vi "Simulator PIM Preset.vi"(8 "error in (no error)":errorcluster, 11 "PIM Configuration":T1={"host IP (localhost)"="localhost", "host Port"=3388, "Model"="", "Serial Number(s)"="", "Calibration Date"=0.0, "Dual Port?"=FALSE, "DeviceNames"=[], "Parameters"={"TX1start"=0.0, "TX1stop"=0.0, "TX1pmax"=0.0, "TX2start"=0.0, "TX2stop"=0.0, "TX2pmax"=0.0, "RXstart"=0.0, "RXstop"=0.0}, "Interface"=enum."PIM Web Engine"} {"Calibration Date" format="%.2f"; "Parameters"."TX2pmax" format="%.1f"; "Parameters"."TX1pmax" format="%.1f"; "Parameters"."RXstop" format="%.1f"; "Parameters"."RXstart" format="%.1f"; "Parameters"."TX2stop" format="%.1f"; "Parameters"."TX2start" format="%.1f"; "Parameters"."TX1stop" format="%.1f"; "Parameters"."TX1start" format="%.1f"}) -> (0 "error out":errorcluster, 2 "Flattened TestSetDef w/Version":string, 3 "TestSetDef":T3={"General"={"ID"=0, "Model"="", "Dual Port?"=FALSE, "Options"="", "Options"={"E"=FALSE, "K"=FALSE, "H"=FALSE, "W"=FALSE, "F"=FALSE}, "Cal File"=path ""}, "Receiver"={"Fstart, MHz"=0.0, "Fstop MHz"=0.0, "Fstep MHz"=0.0, "IF, MHz"=0.0}, "RX Band"={"Fstart, MHz"=0.0, "Fstop MHz"=0.0}, "TX 1"={"Fstart, MHz"=0.0, "Fstop MHz"=0.0, "Pmax, dBm"=0.0, "Pstep, dB"=0.0}, "TX 2"={"Fstart, MHz"=0.0, "Fstop MHz"=0.0, "Pmax, dBm"=0.0, "Pstep, dB"=0.0}, "Low-side?"=TRUE})   [LabVIEW 2011]
uses:
  BPIMCore EXT/HW IO/Test Set Definition.ctl
  PIM Configuration.ctl
  PIM Interface Language.ctl
  Simulator PIM Version.vi
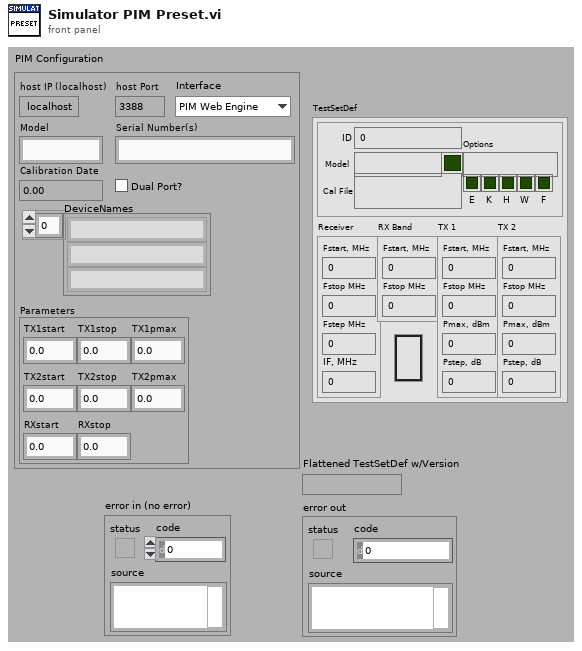
[diagram p1: front panel]
types:
  T1 = typedef "PIM Configuration.ctl" = cluster{"host IP (localhost)":string, "host Port":u16, "Model":string, "Serial Number(s)":string, "Calibration Date":dbl, "Dual Port?":bool, "DeviceNames":string[], "Parameters":cluster{"TX1start":dbl, "TX1stop":dbl, "TX1pmax":dbl, "TX2start":dbl, "TX2stop":dbl, "TX2pmax":dbl, "RXstart":dbl, "RXstop":dbl}, "Interface":T2}
  T2 = typedef "PIM Interface Language.ctl" = enum16{"PIM Web Engine", "PIM HW Engine"}
  T3 = typedef "Test Set Definition.ctl" = cluster{"General":cluster{"ID":u32, "Model":string, "Dual Port?":bool, "Options":string, "Options":cluster{"E":bool, "K":bool, "H":bool, "W":bool, "F":bool}, "Cal File":path}, "Receiver":cluster{"Fstart, MHz":dbl, "Fstop MHz":dbl, "Fstep MHz":dbl, "IF, MHz":dbl}, "RX Band":cluster{"Fstart, MHz":dbl, "Fstop MHz":dbl}, "TX 1":cluster{"Fstart, MHz":dbl, "Fstop MHz":dbl, "Pmax, dBm":dbl, "Pstep, dB":dbl}, "TX 2":cluster{"Fstart, MHz":dbl, "Fstop MHz":dbl, "Pmax, dBm":dbl, "Pstep, dB":dbl}, "Low-side?":bool}
  T4 = typedef "OGAB Version.ctl" = cluster{"Version":string, "Build Number":u32, "Build Date/Time":dbl}
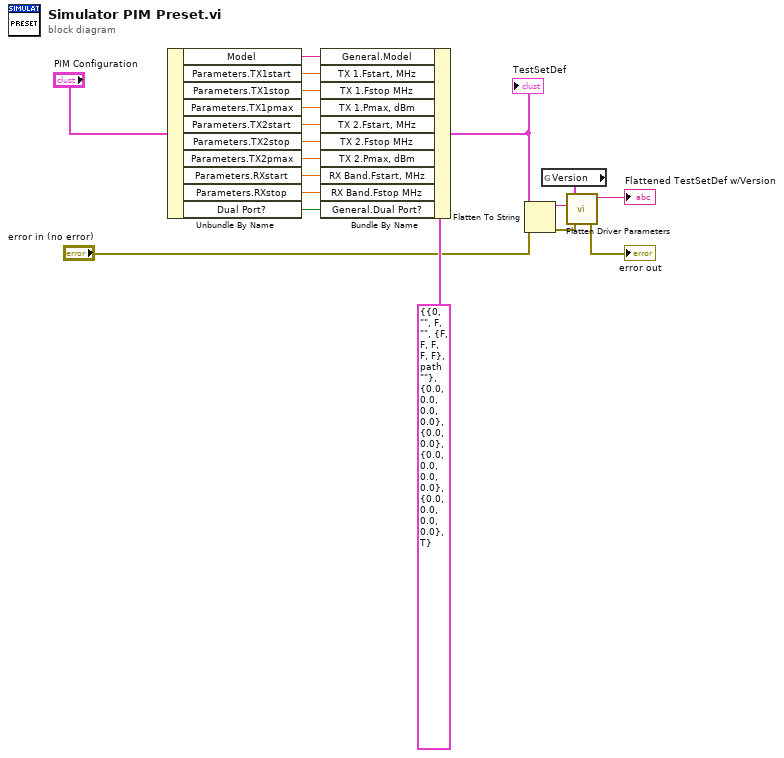
[diagram p0: block diagram]
diagram:
  n1 = Unbundle By Name("PIM Configuration") -> ("Model"=w12:string, "Parameters.TX1start"=w11:dbl, "Parameters.TX1stop"=w10:dbl, "Parameters.TX1pmax"=w9:dbl, "Parameters.TX2start"=w8:dbl, "Parameters.TX2stop"=w7:dbl, "Parameters.TX2pmax"=w6:dbl, "Parameters.RXstart"=w5:dbl, "Parameters.RXstop"=w4:dbl, "Dual Port?"=w1:bool)
  n2 = Bundle By Name(cluster=T3 {"General"={"ID"=0, "Model"="", "Dual Port?"=FALSE, "Options"="", "Options"={"E"=FALSE, "K"=FALSE, "H"=FALSE, "W"=FALSE, "F"=FALSE}, "Cal File"=path ""}, "Receiver"={"Fstart, MHz"=0.0, "Fstop MHz"=0.0, "Fstep MHz"=0.0, "IF, MHz"=0.0}, "RX Band"={"Fstart, MHz"=0.0, "Fstop MHz"=0.0}, "TX 1"={"Fstart, MHz"=0.0, "Fstop MHz"=0.0, "Pmax, dBm"=0.0, "Pstep, dB"=0.0}, "TX 2"={"Fstart, MHz"=0.0, "Fstop MHz"=0.0, "Pmax, dBm"=0.0, "Pstep, dB"=0.0}, "Low-side?"=TRUE} ("TestSetDef"), "General.Model"=w12, "TX 1.Fstart, MHz"=w11, "TX 1.Fstop MHz"=w10, "TX 1.Pmax, dBm"=w9, "TX 2.Fstart, MHz"=w8, "TX 2.Fstop MHz"=w7, "TX 2.Pmax, dBm"=w6, "RX Band.Fstart, MHz"=w5, "RX Band.Fstop MHz"=w4, "General.Dual Port?"=w1) -> (w3:T3)
  "TestSetDef" <- w3
  n3 = Flatten To String(anything=w3, error in (no error)="error in (no error)") -> (data string=w18:string, error out=w16:errorcluster)  [unwired: 3 out]
  n4 = global read "Simulator PIM Version.vi" "Version"() -> (w19:T4)
  n5 = call "Flatten Driver Parameters.vi"("error in (no error)"=w16, "Flattened Driver Parameters (\"\")"=w18, "Driver Version"=w19) -> ("error out"=→"error out":errorcluster, "Flattened Driver Parameters with Version"=→"Flattened TestSetDef w/Version":string)  [unwired: 3 out]
